vi "Set Filter State.vi"(8 "error in (no error)":errorcluster, 10 "Show Action?":bool, 11 "Filter by Is Action In":refnum<class "Filter by Is Action.lvclass">) -> (0 "error out":errorcluster, 3 "Filter by Is Action Out":refnum<class "Filter by Is Action.lvclass">)   [LabVIEW 2020, in "Filter by Is Action.lvclass"]
uses:
  Filter by Is Action.lvclass
  Filter by Is Action.lvclass/Filter by Is Action.ctl
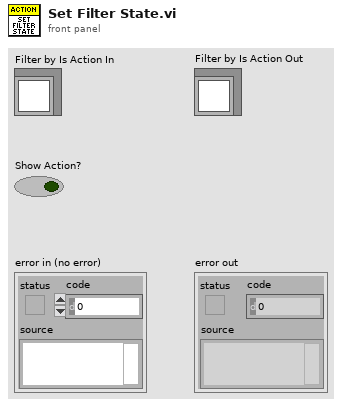
[diagram p1: front panel]
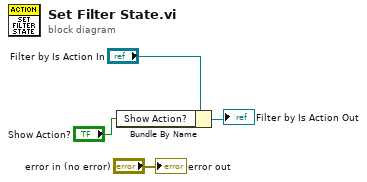
[diagram p0: block diagram]
diagram:
  n1 = Bundle By Name(cluster="Filter by Is Action In", "Show Action?"="Show Action?") -> (→"Filter by Is Action Out":refnum<class "Filter by Is Action.lvclass">)
  "error out" <- "error in (no error)"
